vi "Test 2.vi"(8 "error in (no error)":errorcluster, 11 "Test Case In":refnum<class "Tests Rev3.lvclass">) -> (0 "error out":errorcluster, 3 "Test Case Out":refnum<class "Tests Rev3.lvclass">)   [LabVIEW 2021, in "Tests Rev3.lvclass"]
uses:
  Tests Rev3.lvclass
  Tests Rev3.lvclass/Tests Rev3.ctl
  4993e8ee-a06a-463a-9684-69129f64d5ce.vi
  Proto/Group.lvclass
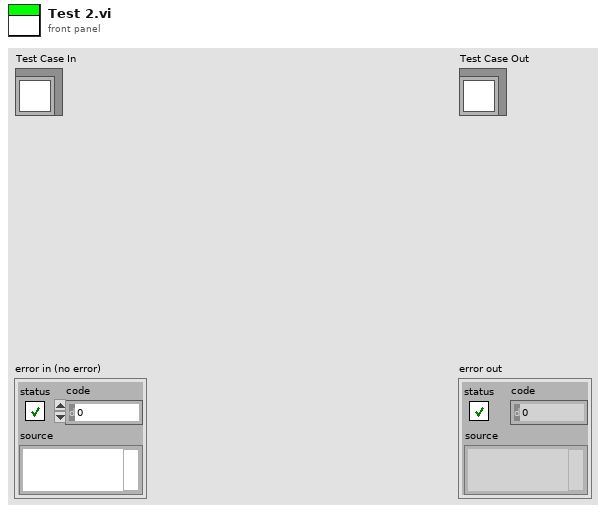
[diagram p1: front panel]
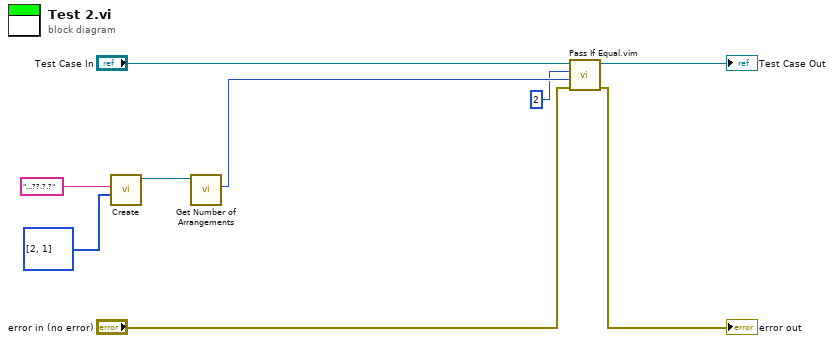
[diagram p0: block diagram]
diagram:
  n1 = call "Create.vi"("Group Sizes"=i64[] [2, 1], "Input"="...??.?.?") -> ("Group Out"=w4:refnum<class "Group.lvclass">)  [unwired: 8 in, 1 out]
  n2 = call "Get Number of Arrangements.vi"("Proto in"=w4) -> ("Arrangements"=w3:u64)  [unwired: 8 in, 2 out]
  n3 = call "Pass If Equal.vim"("error in (no error)"="error in (no error)", "Actual"=w3, "Expected"=u64 2 ("Arrangements"), "LUnit Test Case In"="Test Case In") -> ("error out"=→"error out":errorcluster, "LUnit Test Case Out"=→"Test Case Out":refnum<class "Tests Rev3.lvclass">)  [unwired: 6 in]
